vi "Servo MSMT NR Set RF WFM Parameters.vi"(8 "error in (no error)":errorcluster, 10 "Step In":refnum<k7>, 11 "Servo MSMT in":refnum<class "Servo MSMT.lvclass">) -> (0 "error out":errorcluster, 2 "Step Out":refnum<k7>, 3 "Servo MSMT out":refnum<class "Servo MSMT.lvclass">)   [LabVIEW 2018, in "Servo MSMT.lvlib" / "Servo MSMT.lvclass"]
uses:
  Servo MSMT.lvclass
  Plugins/Measurement Interface.lvlibp/Measurement Interface.lvclass
  C:/Sequence Automation/Plugins/Measurement Interface.lvlibp/Measurement Interface.lvclass
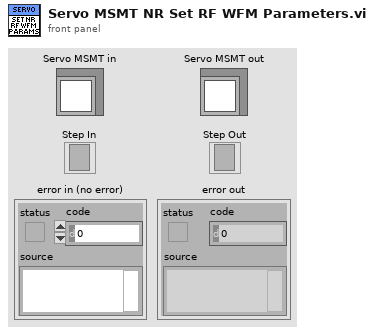
[diagram p1: front panel]
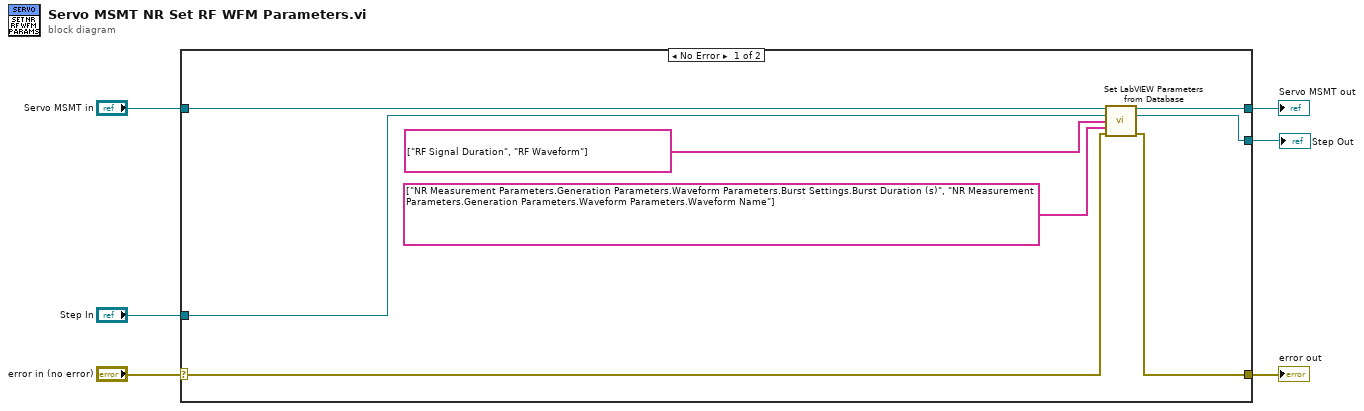
[diagram p0: block diagram]
diagram:
  n1 = case shown="No Error" "error in (no error)" {
    selector: "error in (no error)" -> [w8 w17]
    tunnel: [w7 w17] -> w5
    tunnel: [w12 w16] -> w3
    tunnel: "Servo MSMT in" -> [w14 w16]
    tunnel: [w9 w15] -> w2
    tunnel: "Step In" -> [w11 w15]
    frame No Error {
      n2 = call "Set LabVIEW Parameters from Database.vi"("Measurement Interface in"=w14, "Step In"=w11, "Dictionary Keys"=string[] ["RF Signal Duration", "RF Waveform"], "LabVIEW Parameter Mapping"=string[] ["NR Measurement Parameters.Generation Parameters.Waveform Parameters.Burst Settings.Burst Duration (s)", "NR Measurement Parameters.Generation Parameters.Waveform Parameters.Waveform Name"], "error in (no error)"=w8) -> ("Measurement Interface out"=w12:refnum<class "Servo MSMT.lvclass">, "Step Out"=w9:refnum<k7>, "error out"=w7:errorcluster)  [unwired: 8 in]
    }
    frame Error {
    }
  }
  "error out" <- w5
  "Servo MSMT out" <- w3
  "Step Out" <- w2
